vi "type.remove.vi"(8 "error in":errorcluster, 11 "asset in":refnum<class "asset.lvclass">) -> (0 "error out":errorcluster, 3 "asset out":refnum<class "asset.lvclass">)   [LabVIEW 2020, in "asset.lvclass"]
uses:
  asset.lvclass
  asset.lvclass/asset.ctl
  Nominal Client/Nominal Client.lvclass/Nominal Client.ctl
  Nominal Client/error.vi
  Nominal Client/trace.payload_sent.vi
  Nominal Client/trace.payload_received.vi
  Nominal Client/create.authorization_header.vi
  Nominal Client/error.vi/859f8e04-e495-489b-b5b4-7ac163f56130.vi
  Nominal Client/trace.calling_method.vi
  <vilib>/JDP Science/JDP Science Common Utilities/Trim Whitespace__JDP.vi
  <vilib>/AdvancedString/1D String Array to Delimited String.vi
  Nominal Client/api_token.get.vi
  <vilib>/Utility/libraryn.llb/Get File Extension.vi
  Nominal Client/log_file.write.vi
  <vilib>/JDP Science/JSONtext/Get all Object Items.vi
  <vilib>/Utility/error.llb/Error Cluster From Error Code.vi
  <vilib>/JDP Science/JSONtext/JSON text to Variant.vi
  <vilib>/JDP Science/JSONtext/LVClass Serializer/JSONtext LVClass Serializer.lvclass
  <vilib>/addons/_JKI.lib/REST Client/classes/Response Headers/Response Headers.lvclass
  <vilib>/addons/_JKI.lib/REST Client/classes/REST Client/REST Client.lvclass
  Nominal Client/Nominal Client.lvclass
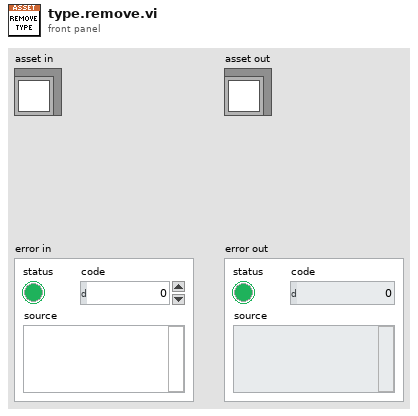
[diagram p1: front panel]
types:
  T1 = typedef "dataScopes.lvlib/links.ctl" = cluster{"URL":string, "Title":string}[]
  T2 = typedef "dataScopes.lvlib/data_scopes.ctl" = T3[]
  T3 = typedef "dataScopes.lvlib/data_scope.ctl" = cluster{"dataScopeName":string, "dataSource":T4, "seriesTags":refnum<class "properties.lvclass">, "offset":T6}
  T4 = typedef "dataScopes.lvlib/data_source.ctl" = cluster{"type":T5, "rid":string}
  T5 = typedef "dataScopes.lvlib/type.ctl" = enum16{"dataset", "connection", "logSet", "video"}
  T6 = typedef "dataScopes.lvlib/offset.ctl" = cluster{"seconds":i32, "nanos":i32, "picos":i32}
  T7 = cluster{"rid":string, "title":string, "properties":refnum<class "properties.lvclass">, "labels":refnum<class "labels.lvclass">, "Links":T1, "datascopes":T2, "createdAt":timestamp, "updatedAt":timestamp, "attachments":refnum<class "labels.lvclass">, "isStaged":bool, "isArchived":bool, "description":string, "createdBy":string, "type":string}
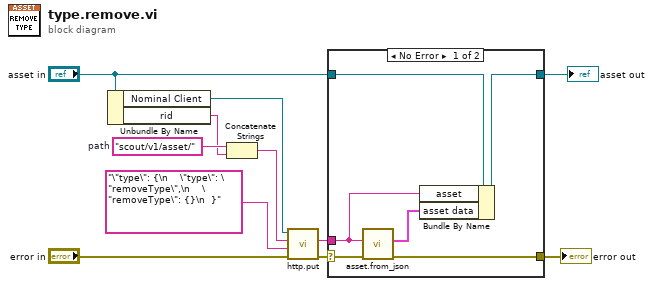
[diagram p0: block diagram]
diagram:
  w10 = "scout/v1/asset/"  # path
  n1 = Unbundle By Name("asset in") -> ("Nominal Client"=w11:refnum<class "Nominal Client.lvclass">, "rid"=w8:string)
  n2 = Concatenate Strings(w10, w8) -> (w9:string)
  n3 = call "http.put.vi"("error in"="error in", "Body"="\"type\": {\n    \"type\": \"removeType\",\n    \"removeType\": {}\n  }", "Path"=w9, "Nominal Client in"=w11) -> ("error out"=w7:errorcluster, "Response"=w4:string)  [unwired: 4 in, 2 out]
  n4 = case shown="No Error" w7 {
    selector: w7 -> [w17 w19]
    tunnel: [w16 w19] -> w6
    tunnel: "asset in" -> [w15 w18]
    tunnel: w4 -> [w13 _]
    tunnel: [w12 w18] -> w3
    frame No Error {
      n5 = call "asset.from_json.vi"("error in"=w17, "asset"=w13) -> ("error out"=w16:errorcluster, "Asset Data"=w14:T7)  [unwired: 8 in]
      n6 = Bundle By Name(cluster=w15, "asset"=w13, "asset data"=w14) -> (w12:refnum<class "asset.lvclass">)
    }
    frame Error {
    }
  }
  "asset out" <- w3
  "error out" <- w6
